vi "Begin.vi"(8 "error in":errorcluster) -> (0 "error out":errorcluster)   [LabVIEW 2015]
doc: "Called before other user functions, this VI is expected to open initial I/O refnums, load in file data, and do all program initialization. Notice that the <B>error out</B> terminal is simply used for data flow. Wiring it to other structures or subVIs ensures that this VI runs first."
uses:
  <vilib>/Rock Robotics/WPI/DriverStation/WPI_DriverStationRobotMode2.ctl
  <vilib>/Rock Robotics/WPI/Joystick/WPI_JoystickDeviceEnum.ctl
  <vilib>/Rock Robotics/WPI/CAN/TalonSRX/WPI_CANTalonSRX_APIControlMode.ctl
  <vilib>/Rock Robotics/SystemInterfaces/i2clib/i2c_bus.ctl
  <vilib>/Rock Robotics/SystemInterfaces/DIO/FPGA_DIOChannel.ctl
  <vilib>/Rock Robotics/WPI/Solenoid/WPI_SolenoidChannel.ctl
  <vilib>/Rock Robotics/WPI/SafetyOutput/WPI_SafetyOutputConfigMenu.ctl
  Robot Global Data.vi
  <vilib>/Rock Robotics/Network Tables/NT Write String Array.vi
  <vilib>/Rock Robotics/WPI/RobotDrive/WPI_RobotDriveOpen2MotorWithCANTalonSRX.vi
  <vilib>/Rock Robotics/WPI/MotorControl/WPI_MotorControlOpenCANTalonSRX.vi
  <vilib>/Rock Robotics/WPI/Solenoid/WPI_SolenoidOpenDouble.vi
  <vilib>/Rock Robotics/WPI/MotorControl/WPI_MotorControlOpen Talon.vi
panel:
  out "i2c Error":errorcluster
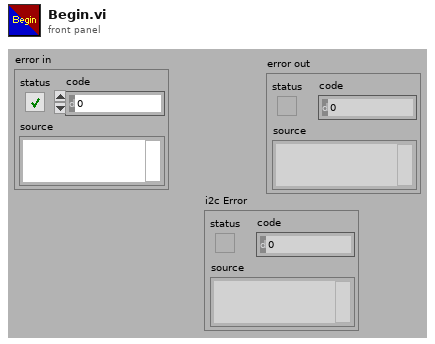
[diagram p1: front panel]
types:
  T1 = typedef "WPI_SafetyOutputConfigMenu.ctl" = enum16{"Enable", "Disable"}
  T2 = typedef "WPI_JoystickDeviceEnum.ctl" = enum16{"USB 0", "USB 1", "USB 2", "USB 3", "USB 4", "USB 5"}
  T3 = typedef "WPI_SolenoidChannel.ctl" = enum8{"Solenoid 0", "Solenoid 1", "Solenoid 2", "Solenoid 3", "Solenoid 4", "Solenoid 5", "Solenoid 6", "Solenoid 7", "Invalid"}
  T4 = typedef "FPGA_DIOChannel.ctl" = enum8{"DIO 0", "DIO 1", "DIO 2", "DIO 3", "DIO 4", "DIO 5", "DIO 6", "DIO 7", "DIO 8", "DIO 9", "DIO MXP 0", "DIO MXP 1", "DIO MXP 2", "DIO MXP 3", "DIO MXP 4", "DIO MXP 5", "DIO MXP 6", "DIO MXP 7", "DIO MXP 8", "DIO MXP 9", "DIO MXP 10", "DIO MXP 11", "DIO MXP 12", "DIO MXP 13", "DIO MXP 14", "DIO MXP 15", "Invalid"}
  T5 = typedef "i2c_bus.ctl" = enum16{"I2C On-Board", "I2C MXP", "Invalid"}
  T6 = typedef "WPI_CANTalonSRX_APIControlMode.ctl" = enum8{"Percent VBus", "Speed", "Position", "Slave", "Unchanged / Invalid", "Voltage Compensation", "Current", "Motion Profile"}
  T7 = typedef "WPI_DriverStationRobotMode2.ctl" = enum16{"Autonomous Disabled", "Autonomous Enabled", "Teleop Disabled", "Teleop Enabled", "Disconnected", "Finish", "Test Disabled", "Test Enabled", "Emergency Stopped"}
  T8 = typedef "WPI_JoystickDevRef.ctl" = cluster{"Device":T2}
  T9 = typedef "WPI_RobotDriveDevRef.ctl" = cluster{"DevStatus":errorcluster, "Motors[]":T10[], "Square Inputs":bool, "Max Output":dbl}
  T10 = typedef "WPI_MotorControlDeviceRef.ctl" = cluster{"DeviceStatus":errorcluster, "Type":T11, "PWM":cluster{"PWM Channel":T12, "DeadBand":T13}, "CAN":cluster{"Device Number":u8, "Control Mode":T14, "Semaphore":T15, "Max Vout":dbl, "TalonSRX Control Mode":T6}, "Invert":bool}
  T11 = typedef "WPI_MotorControlType.ctl" = enum16{"PWM", "CAN", "CANTalonSRX"}
  T12 = typedef "FPGA_DIOPWMChannel.ctl" = enum8{"PWM 0", "PWM 1", "PWM 2", "PWM 3", "PWM 4", "PWM 5", "PWM 6", "PWM 7", "PWM 8", "PWM 9", "PWM MXP 0", "PWM MXP 1", "PWM MXP 2", "PWM MXP 3", "PWM MXP 4", "PWM MXP 5", "PWM MXP 6", "PWM MXP 7", "PWM MXP 8", "PWM MXP 9", "Invalid"}
  T13 = typedef "WPI_PWMDeadband.ctl" = cluster{"Name":string, "maxPositivePwm":i32, "minPositivePwm":i32, "centerPwm":i32, "maxNegativePwm":i32, "minNegativePwm":i32, "angularRange":u16}
  T14 = typedef "WPI_CANJaguar_ControlMode.ctl" = enum8{"Percent VBus", "Current", "Speed", "Position", "Voltage"}
  T15 = typedef "Semaphore RefNum" = refnum<k1>
  T16 = typedef "WPI_DigitalInputDevRef.ctl" = cluster{"DevStatus":errorcluster, "DIO Channel":T4}
  T17 = typedef "WPI_SolenoidDevRef.ctl" = cluster{"DevStatus":errorcluster, "Pneumatics Control Module":u8, "Forward Solenoid Channel":T3, "Reverse Solenoid Channel":T3}
  T18 = typedef "WPI_I2CDevRef.ctl" = cluster{"DevStatus":errorcluster, "Device Address":u8, "Handle":i32, "I2C Bus":T5}
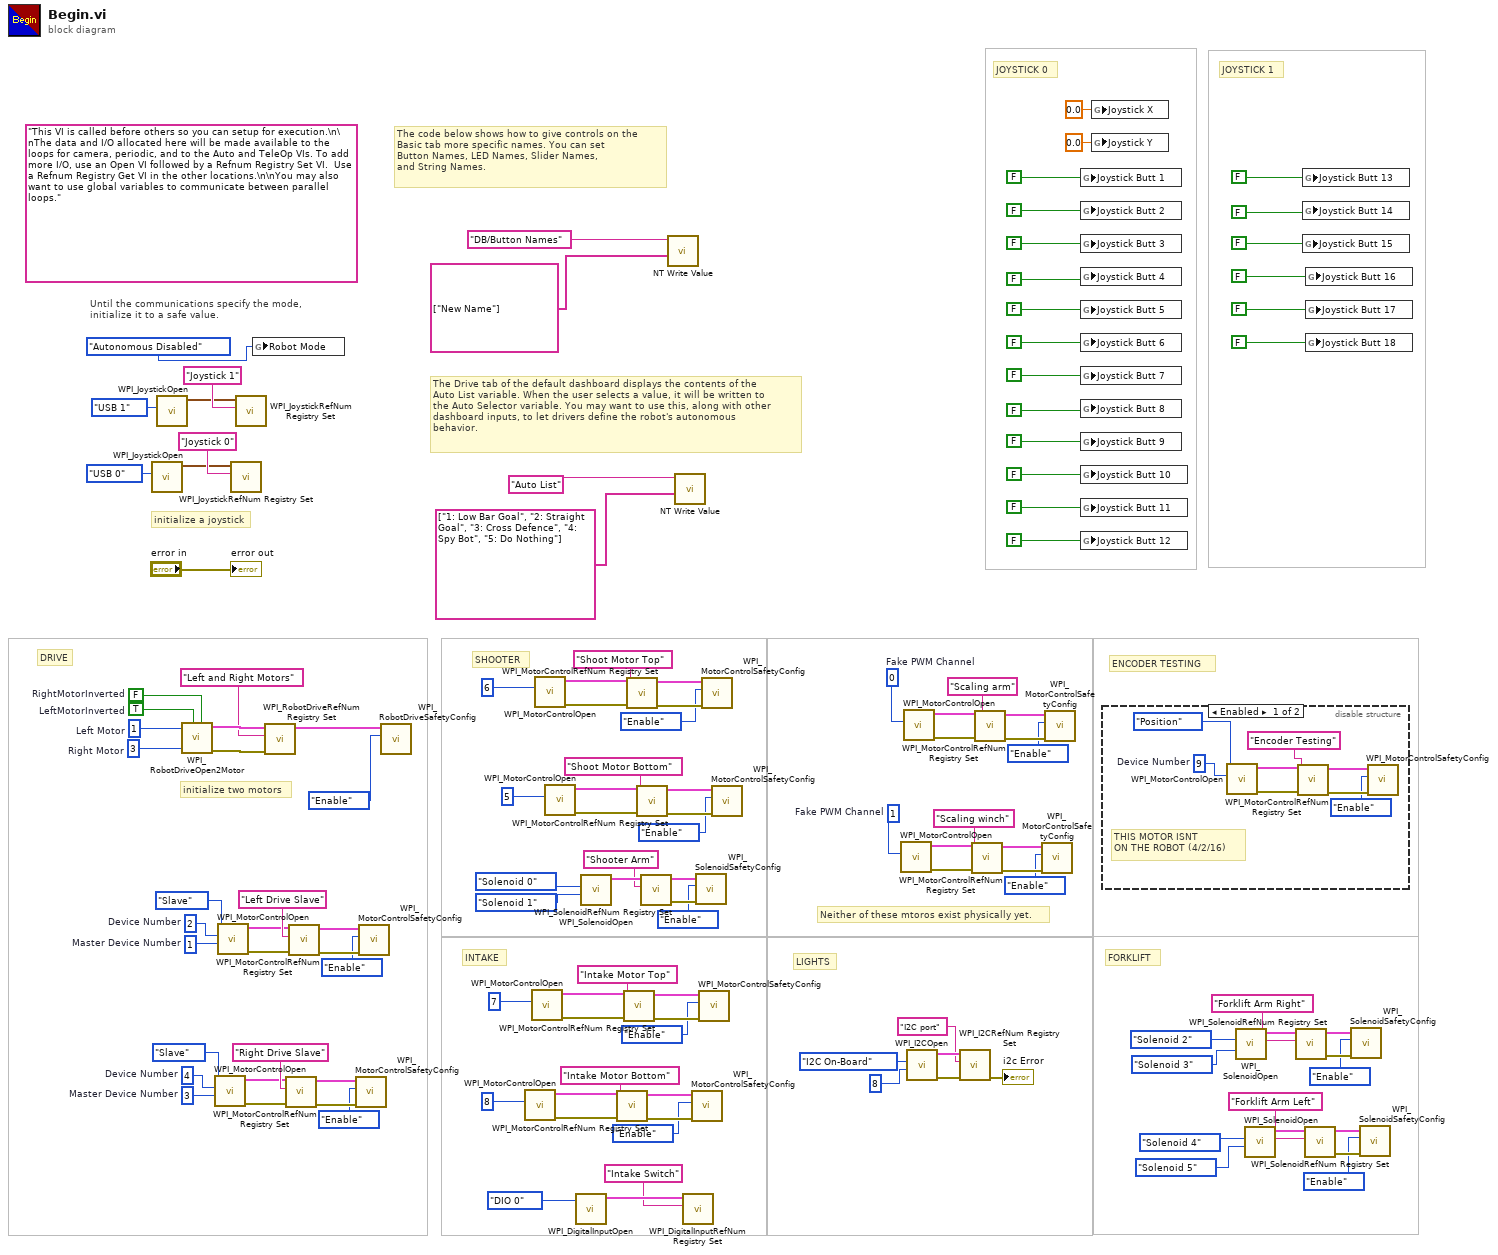
[diagram p0: block diagram]
diagram:
  w7 = u8 1  # Fake PWM Channel
  w14 = u8 0  # Fake PWM Channel
  w85 = u8 3  # Master Device Number
  w92 = u8 4  # Device Number
  w94 = u8 1  # Master Device Number
  w101 = u8 3  # Right Motor
  w102 = u8 1  # Left Motor
  w103 = u8 2  # Device Number
  (unwired) "This VI is called before others so you can setup for execution.\n\nThe data and I/O allocated here will be made available to the loops for camera, periodic, and to the Auto and TeleOp VIs. To add more I/O, use an Open VI followed by a Refnum Registry Set VI.  Use a Refnum Registry Get VI in the other locations.\n\nYou may also want to use global variables to communicate between parallel loops."
  w130 = TRUE  # LeftMotorInverted
  w131 = FALSE  # RightMotorInverted
  # "Neither of these mtoros exist physically yet."
  # "JOYSTICK 1"
  # "JOYSTICK 0"
  # "DRIVE"
  # "FORKLIFT"
  # "ENCODER TESTING"
  # "LIGHTS"
  # "INTAKE"
  # "SHOOTER"
  # "The Drive tab of the default dashboard displays the contents of the\nAuto List variable. When the user selects a value, it will be written to\nthe Auto Selector variable. You may want to use this, along with other\ndashboard inputs, to let drivers define the robot's autonomous\nbehavior."
  # "The code below shows how to give controls on the\nBasic tab more specific names. You can set\nButton Names, LED Names, Slider Names,\nand String Names."
  # "initialize a joystick"
  # "Until the communications specify the mode,\ninitialize it to a safe value."
  # "initialize two motors"
  n1 = call <vilib>:"WPI_JoystickOpen.vi"("JoystickDevice"=WPI_JoystickDeviceEnum."USB 0") -> ("JoystickDevRef"=w123:T8)  [unwired: 10 in]
  n2 = call <vilib>:"WPI_JoystickOpen.vi"("JoystickDevice"=WPI_JoystickDeviceEnum."USB 1") -> ("JoystickDevRef"=w22:T8)  [unwired: 10 in]
  n3 = call-poly <vilib>:"WPI_RobotDriveOpen2Motor.vi"("Right Motor Inverted"=w131, "Left Motor Inverted"=w130, "Right Motor"=w101, "Left Motor"=w102) -> ("error out"=w127:errorcluster, "RobotDriveDevRef"=w129:T9)  [unwired: 1 in, 5 out]
  n4 = call-poly <vilib>:"WPI_MotorControlOpen.vi"("Master Device Number"=w85, "Device Number"=w92, "Control Mode"=WPI_CANTalonSRX_APIControlMode."Slave") -> ("error out"=w89:errorcluster, "MotorControlDeviceRef"=w90:T10)  [unwired: 7 in]
  n5 = call-poly <vilib>:"WPI_MotorControlOpen.vi"("Master Device Number"=w94, "Device Number"=w103, "Control Mode"=WPI_CANTalonSRX_APIControlMode."Slave") -> ("error out"=w98:errorcluster, "MotorControlDeviceRef"=w99:T10)  [unwired: 7 in]
  n6 = call <vilib>:"WPI_JoystickRefNum Registry Set.vi"("refnum name"="Joystick 0", "JoystickDevRef"=w123) -> ()  [unwired: 8 in, 2 out]
  n7 = call <vilib>:"WPI_JoystickRefNum Registry Set.vi"("refnum name"="Joystick 1", "JoystickDevRef"=w22) -> ()  [unwired: 8 in, 2 out]
  n8 = global write "Robot Global Data.vi" "Robot Mode"(WPI_DriverStationRobotMode2."Autonomous Disabled" ("Robot Mode")) -> ()
  n9 = call <vilib>:"WPI_RobotDriveRefNum Registry Set.vi"("error in (no error)"=w127, "refnum name"="Left and Right Motors", "RobotDriveDevRef"=w129) -> ("RobotDriveDevRef"=w126:T9)  [unwired: 1 in, 7 out]
  n10 = call <vilib>:"WPI_MotorControlRefNum Registry Set.vi"("error in (no error)"=w89, "refnum name"="Right Drive Slave", "MotorControlDevRef"=w90) -> ("error out"=w88:errorcluster, "MotorControlDevRef"=w87:T10)  [unwired: 7 in]
  n11 = call <vilib>:"WPI_MotorControlRefNum Registry Set.vi"("error in (no error)"=w98, "refnum name"="Left Drive Slave", "MotorControlDevRef"=w99) -> ("error out"=w97:errorcluster, "MotorControlDevRef"=w96:T10)  [unwired: 7 in]
  n12 = call <vilib>:"WPI_MotorControlSafetyConfig.vi"("error in (no error)"=w88, "mode"=WPI_SafetyOutputConfigMenu."Enable", "MotorControlDevRef"=w87) -> ()  [unwired: 7 in, 2 out]
  n13 = call <vilib>:"WPI_MotorControlSafetyConfig.vi"("error in (no error)"=w97, "mode"=WPI_SafetyOutputConfigMenu."Enable", "MotorControlDevRef"=w96) -> ()  [unwired: 7 in, 2 out]
  n14 = call <vilib>:"WPI_RobotDriveSafetyConfig.vi"("mode"=WPI_SafetyOutputConfigMenu."Enable", "RobotDriveDevRef"=w126) -> ()  [unwired: 8 in, 2 out]
  n15 = call-poly <vilib>:"WPI_MotorControlOpen.vi"("Device Number"=u8 8) -> ("error out"=w60:errorcluster, "MotorControlDeviceRef"=w59:T10)  [unwired: 9 in]
  n16 = call-poly <vilib>:"WPI_MotorControlOpen.vi"("Device Number"=u8 7) -> ("error out"=w53:errorcluster, "MotorControlDeviceRef"=w52:T10)  [unwired: 9 in]
  n17 = call-poly <vilib>:"WPI_MotorControlOpen.vi"("Device Number"=u8 6) -> ("error out"=w115:errorcluster, "MotorControlDeviceRef"=w114:T10)  [unwired: 9 in]
  n18 = call-poly <vilib>:"WPI_MotorControlOpen.vi"("Device Number"=u8 5) -> ("error out"=w109:errorcluster, "MotorControlDeviceRef"=w108:T10)  [unwired: 9 in]
  n19 = call <vilib>:"WPI_DigitalInputOpen.vi"("DIO Channel"=FPGA_DIOChannel."DIO 0") -> ("DigitalInputDevRef"=w77:T16)  [unwired: 9 in, 1 out]
  n20 = call-poly <vilib>:"WPI_SolenoidOpen.vi"("Reverse Solenoid Channel"=WPI_SolenoidChannel."Solenoid 1", "Forward Solenoid Channel"=WPI_SolenoidChannel."Solenoid 0" ("Solenoid Channel")) -> ("SolenoidDevRef"=w40:T17)  [unwired: 8 in, 1 out]
  n21 = call <vilib>:"WPI_MotorControlRefNum Registry Set.vi"("error in (no error)"=w60, "refnum name"="Intake Motor Bottom", "MotorControlDevRef"=w59) -> ("error out"=w56:errorcluster, "MotorControlDevRef"=w57:T10)  [unwired: 7 in]
  n22 = call <vilib>:"WPI_MotorControlRefNum Registry Set.vi"("error in (no error)"=w53, "refnum name"="Intake Motor Top", "MotorControlDevRef"=w52) -> ("error out"=w49:errorcluster, "MotorControlDevRef"=w50:T10)  [unwired: 7 in]
  n23 = call <vilib>:"WPI_MotorControlRefNum Registry Set.vi"("error in (no error)"=w115, "refnum name"="Shoot Motor Top", "MotorControlDevRef"=w114) -> ("error out"=w111:errorcluster, "MotorControlDevRef"=w112:T10)  [unwired: 7 in]
  n24 = call <vilib>:"WPI_MotorControlRefNum Registry Set.vi"("error in (no error)"=w109, "refnum name"="Shoot Motor Bottom", "MotorControlDevRef"=w108) -> ("error out"=w105:errorcluster, "MotorControlDevRef"=w106:T10)  [unwired: 7 in]
  n25 = call <vilib>:"WPI_SolenoidRefNum Registry Set.vi"("refnum name"="Shooter Arm", "SolenoidDevRef"=w40) -> ("error out"=w39:errorcluster, "SolenoidDevRef"=w38:T17)  [unwired: 8 in]
  n26 = call-poly <vilib>:"NT Write Value.vi"("String Array"=string[] ["New Name"], "Name"="DB/Button Names") -> ()  [unwired: 9 in, 1 out]
  n27 = call-poly <vilib>:"NT Write Value.vi"("String Array"=string[] ["1: Low Bar Goal", "2: Straight Goal", "3: Cross Defence", "4: Spy Bot", "5: Do Nothing"], "Name"="Auto List") -> ()  [unwired: 9 in, 1 out]
  n28 = call <vilib>:"WPI_DigitalInputRefNum Registry Set.vi"("refnum name"="Intake Switch", "DigitalInputDevRef"=w77) -> ()  [unwired: 8 in, 2 out]
  n29 = call <vilib>:"WPI_MotorControlSafetyConfig.vi"("error in (no error)"=w56, "mode"=WPI_SafetyOutputConfigMenu."Enable", "MotorControlDevRef"=w57) -> ()  [unwired: 7 in, 2 out]
  n30 = call <vilib>:"WPI_SolenoidSafetyConfig.vi"("error in (no error)"=w39, "mode"=WPI_SafetyOutputConfigMenu."Enable", "SolenoidDevRef"=w38) -> ()  [unwired: 7 in, 2 out]
  n31 = call <vilib>:"WPI_MotorControlSafetyConfig.vi"("error in (no error)"=w49, "mode"=WPI_SafetyOutputConfigMenu."Enable", "MotorControlDevRef"=w50) -> ()  [unwired: 7 in, 2 out]
  n32 = call <vilib>:"WPI_MotorControlSafetyConfig.vi"("error in (no error)"=w111, "mode"=WPI_SafetyOutputConfigMenu."Enable", "MotorControlDevRef"=w112) -> ()  [unwired: 7 in, 2 out]
  n33 = call <vilib>:"WPI_MotorControlSafetyConfig.vi"("error in (no error)"=w105, "mode"=WPI_SafetyOutputConfigMenu."Enable", "MotorControlDevRef"=w106) -> ()  [unwired: 7 in, 2 out]
  n34 = call-poly <vilib>:"WPI_MotorControlOpen.vi"("PWM Channel"=w7) -> ("error out"=w4:errorcluster, "MotorControlDeviceRef"=w5:T10)  [unwired: 9 in]
  n35 = call-poly <vilib>:"WPI_MotorControlOpen.vi"("PWM Channel"=w14) -> ("error out"=w11:errorcluster, "MotorControlDeviceRef"=w12:T10)  [unwired: 9 in]
  n36 = call <vilib>:"WPI_I2COpen.vi"("Device Address"=u8 8, "I2C Bus"=i2c_bus."I2C On-Board") -> ("error out"=w79:errorcluster, "I2CDevRef"=w83:T18)  [unwired: 8 in]
  n37 = call <vilib>:"WPI_I2CRefNum Registry Set.vi"("error in (no error)"=w79, "refnum name"="I2C port", "I2CDevRef"=w83) -> ("error out"=→"i2c Error":errorcluster)  [unwired: 7 in, 1 out]
  n38 = call <vilib>:"WPI_MotorControlRefNum Registry Set.vi"("error in (no error)"=w4, "refnum name"="Scaling winch", "MotorControlDevRef"=w5) -> ("error out"=w3:errorcluster, "MotorControlDevRef"=w2:T10)  [unwired: 7 in]
  n39 = call <vilib>:"WPI_MotorControlRefNum Registry Set.vi"("error in (no error)"=w11, "refnum name"="Scaling arm", "MotorControlDevRef"=w12) -> ("error out"=w10:errorcluster, "MotorControlDevRef"=w9:T10)  [unwired: 7 in]
  n40 = call <vilib>:"WPI_MotorControlSafetyConfig.vi"("error in (no error)"=w3, "mode"=WPI_SafetyOutputConfigMenu."Enable", "MotorControlDevRef"=w2) -> ()  [unwired: 7 in, 2 out]
  n41 = call <vilib>:"WPI_MotorControlSafetyConfig.vi"("error in (no error)"=w10, "mode"=WPI_SafetyOutputConfigMenu."Enable", "MotorControlDevRef"=w9) -> ()  [unwired: 7 in, 2 out]
  n42 = global write "Robot Global Data.vi" "Joystick Butt 1"(FALSE) -> ()
  n43 = global write "Robot Global Data.vi" "Joystick Butt 2"(FALSE) -> ()
  n44 = global write "Robot Global Data.vi" "Joystick Butt 3"(FALSE) -> ()
  n45 = global write "Robot Global Data.vi" "Joystick Butt 4"(FALSE) -> ()
  n46 = global write "Robot Global Data.vi" "Joystick Butt 5"(FALSE) -> ()
  n47 = global write "Robot Global Data.vi" "Joystick Butt 6"(FALSE) -> ()
  n48 = global write "Robot Global Data.vi" "Joystick Butt 7"(FALSE) -> ()
  n49 = global write "Robot Global Data.vi" "Joystick Butt 8"(FALSE) -> ()
  n50 = global write "Robot Global Data.vi" "Joystick Butt 9"(FALSE) -> ()
  n51 = global write "Robot Global Data.vi" "Joystick Butt 10"(FALSE) -> ()
  n52 = global write "Robot Global Data.vi" "Joystick Butt 11"(FALSE) -> ()
  n53 = global write "Robot Global Data.vi" "Joystick Butt 12"(FALSE) -> ()
  n54 = global write "Robot Global Data.vi" "Joystick X"(0.0 ("Joystick X")) -> ()
  n55 = global write "Robot Global Data.vi" "Joystick Y"(0.0 ("Joystick Y")) -> ()
  n56 = disable-structure shown="Enabled" {
    frame Enabled {
      w139 = u8 9  # Device Number
      # "THIS MOTOR ISNT\nON THE ROBOT (4/2/16)"
      n57 = call-poly <vilib>:"WPI_MotorControlOpen.vi"("Device Number"=w139, "Control Mode"=WPI_CANTalonSRX_APIControlMode."Position") -> ("error out"=w136:errorcluster, "MotorControlDeviceRef"=w137:T10)  [unwired: 8 in]
      n58 = call <vilib>:"WPI_MotorControlRefNum Registry Set.vi"("error in (no error)"=w136, "refnum name"="Encoder Testing", "MotorControlDevRef"=w137) -> ("error out"=w135:errorcluster, "MotorControlDevRef"=w134:T10)  [unwired: 7 in]
      n59 = call <vilib>:"WPI_MotorControlSafetyConfig.vi"("error in (no error)"=w135, "mode"=WPI_SafetyOutputConfigMenu."Enable", "MotorControlDevRef"=w134) -> ()  [unwired: 7 in, 2 out]
    }
    frame Disabled {
    }
  }
  n60 = call-poly <vilib>:"WPI_SolenoidOpen.vi"("Reverse Solenoid Channel"=WPI_SolenoidChannel."Solenoid 3", "Forward Solenoid Channel"=WPI_SolenoidChannel."Solenoid 2" ("Solenoid Channel")) -> ("SolenoidDevRef"=w45:T17)  [unwired: 8 in, 1 out]
  n61 = call-poly <vilib>:"WPI_SolenoidOpen.vi"("Reverse Solenoid Channel"=WPI_SolenoidChannel."Solenoid 5" ("Forward Solenoid Channel"), "Forward Solenoid Channel"=WPI_SolenoidChannel."Solenoid 4" ("Solenoid Channel")) -> ("SolenoidDevRef"=w35:T17)  [unwired: 8 in, 1 out]
  n62 = call <vilib>:"WPI_SolenoidRefNum Registry Set.vi"("refnum name"="Forklift Arm Right", "SolenoidDevRef"=w45) -> ("error out"=w44:errorcluster, "SolenoidDevRef"=w43:T17)  [unwired: 8 in]
  n63 = global write "Robot Global Data.vi" "Joystick Butt 13"(FALSE) -> ()
  n64 = global write "Robot Global Data.vi" "Joystick Butt 14"(FALSE) -> ()
  n65 = global write "Robot Global Data.vi" "Joystick Butt 15"(FALSE) -> ()
  n66 = call <vilib>:"WPI_SolenoidRefNum Registry Set.vi"("refnum name"="Forklift Arm Left", "SolenoidDevRef"=w35) -> ("error out"=w34:errorcluster, "SolenoidDevRef"=w33:T17)  [unwired: 8 in]
  n67 = global write "Robot Global Data.vi" "Joystick Butt 16"(FALSE) -> ()
  n68 = global write "Robot Global Data.vi" "Joystick Butt 17"(FALSE) -> ()
  n69 = global write "Robot Global Data.vi" "Joystick Butt 18"(FALSE) -> ()
  n70 = call <vilib>:"WPI_SolenoidSafetyConfig.vi"("error in (no error)"=w44, "mode"=WPI_SafetyOutputConfigMenu."Enable", "SolenoidDevRef"=w43) -> ()  [unwired: 7 in, 2 out]
  n71 = call <vilib>:"WPI_SolenoidSafetyConfig.vi"("error in (no error)"=w34, "mode"=WPI_SafetyOutputConfigMenu."Enable", "SolenoidDevRef"=w33) -> ()  [unwired: 7 in, 2 out]
  "error out" <- "error in"
